vi "TRDU_ADRESSAGE.vi"(8 "errin":errorcluster, 11 "Go?":bool) -> (0 "errout":errorcluster, 2 "Branche":dbl=1.0, 3 "Addressé?":bool)   [LabVIEW 2020]
uses:
  <userlib>/PCAN Basic/Controls/BaudrateEenum.ctl
  <userlib>/PCAN Basic/Controls/Channel.ctl
  OP500/VG/VG_branche.vi
  <userlib>/PCAN Basic/PCANBasic.lvlib
  <userlib>/Alex_Peak_lib/PEAK_lib_ALEX.lvlib
panel:
  out "OBJ":u8[](array[numeric])
  out "CAN":u8[](array[numeric])
  # "READ FROM CAN"
  # "OBJECTIVE TO PASS"
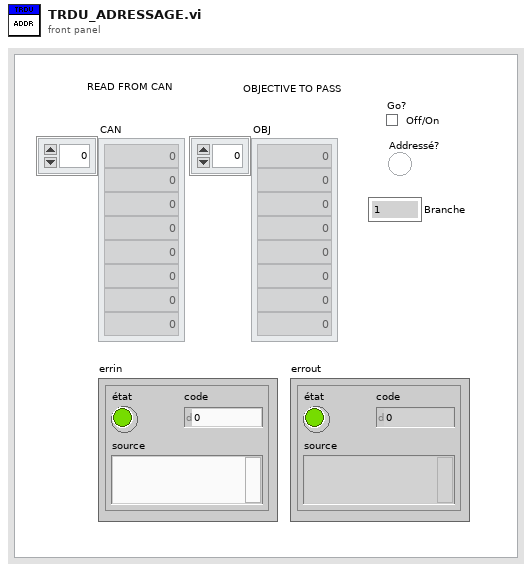
[diagram p1: front panel]
types:
  T1 = typedef "PCANBasic.lvlib/Channel.ctl" = enum16{"PCAN_NONEBUS", "not used1", "not used2", "not used3", "not used4", "not used5", "not used6", "not used7", "not used8", "not used9", "not used10", "not used11", "not used12", "not used13", "not used14", "not used15", "not used16", "not used17", "not used18", "not used19", "not used20", "not used21", "not used22", "not used23", "not used24", "not used25", "not used26", "not used27", "not used28", "not used29", "not used30", "not used31", "not used32", "PCAN_ISABUS1", "PCAN_ISABUS2", "PCAN_ISABUS3", "PCAN_ISABUS4", "PCAN_ISABUS5", "PCAN_ISABUS6", "PCAN_ISABUS7", "PCAN_ISABUS8", "not used41", "not used42", "not used43", "not used44", "not used45", "not used46", "not used47", "not used48", "PCAN_DNGBUS1", "not used50", "not used51", "not used52", "not used53", "not used54", "not used55", "not used56", "not used57", "not used58", "not used59", "not used60", "not used61", "not used62", "not used63", "not used64", "PCAN_PCIBUS1", "PCAN_PCIBUS2", "PCAN_PCIBUS3", "PCAN_PCIBUS4", "PCAN_PCIBUS5", "PCAN_PCIBUS6", "PCAN_PCIBUS7", "PCAN_PCIBUS8", "not used73", "not used74", "not used75", "not used76", "not used77", "not used78", "not used79", "not used80", "PCAN_USBBUS1", "PCAN_USBBUS2", "PCAN_USBBUS3", "PCAN_USBBUS4", "PCAN_USBBUS5", "PCAN_USBBUS6", "PCAN_USBBUS7", "PCAN_USBBUS8", "Not used89", "Not used90", "Not used91", "Not used92", "Not used93", "Not used94", "Not used95", "Not used96", "PCAN_PCCBUS1", "PCAN_PCCBUS2"}
  T2 = typedef "PCANBasic.lvlib/BaudrateEenum.ctl" = enum16{"CAN_Baud_1M", "CAN_Baud_800K", "CAN_BAUD_500K", "CAN_BAUD_250K", "CAN_BAUD_125K", "CAN_BAUD_100K", "CAN_BAUD_95K", "CAN_BAUD_83K", "CAN_BAUD_50K", "CAN_BAUD_47K", "CAN_BAUD_33K", "CAN_BAUD_20K", "CAN_BAUD_10K", "CAN_BAUD_5K", "User Baudrate"}
  T3 = cluster{"ID":u32, "MSGTYPE":u8, "LEN":u8, "DATA[0]":u8, "DATA[1]":u8, "DATA[2]":u8, "DATA[3]":u8, "DATA[4]":u8, "DATA[5]":u8, "DATA[6]":u8, "DATA[7]":u8}
  T4 = cluster{"DATA[0]":u8, "DATA[1]":u8, "DATA[2]":u8, "DATA[3]":u8, "DATA[4]":u8, "DATA[5]":u8, "DATA[6]":u8, "DATA[7]":u8}
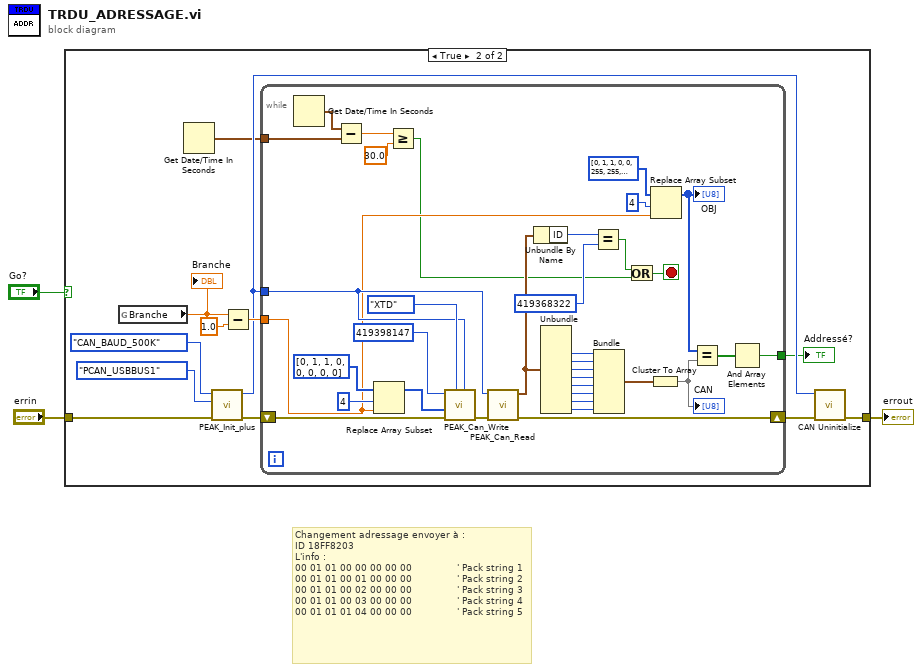
[diagram p0: block diagram]
diagram:
  # "Changement adressage envoyer à :\nID 18FF8203 \nL'info :\n00 01 01 00 00 00 00 00               ' Pack string 1\n00 01 01 00 01 00 00 00               ' Pack string 2\n00 01 01 00 02 00 00 00               ' Pack string 3\n00 01 01 00 03 00 00 00               ' Pack string 4\n00 01 01 01 04 00 00 00               ' Pack string 5"
  n1 = case shown="True" "Go?" {
    tunnel: "errin" -> [w4 w16]
    tunnel: [w4 w8] -> w2
    frame False {
    }
    frame True {
      n2 = global read "VG_branche.vi" "Branche"() -> (w12:dbl)
      "Branche" <- w12
      n3 = Get Date/Time In Seconds() -> (seconds since 1Jan1904=w5:timestamp)
      n4 = call <userlib>:"PEAK_Init_plus.vi"("errin"=w16, "Channel"=Channel."PCAN_USBBUS1", "BTR0BTR1"=BaudrateEenum."CAN_BAUD_500K") -> ("errout"=w13:errorcluster, "Channel out"=w7:T1)  [unwired: 7 in]
      n5 = Subtract(x=w12, y=1.0) -> (x-y=w10:dbl)
      n6 = while {
        tunnel: w10 -> [w38]
        tunnel: w7 -> [w43]
        shift-right: [w44] -> w9
        shift-left: w13 -> [w50]
        tunnel: [w24] -> w6
        tunnel: w5 -> [w20]
        stop <- w22 stop-if-true
        n7 = Get Date/Time In Seconds() -> (seconds since 1Jan1904=w21:timestamp)
        n8 = Subtract(x=w21, y=w20) -> (x-y=w19:dbl)
        n9 = Replace Array Subset(array=u8[] [0, 1, 1, 0, 0, 0, 0, 0] ("CAN Data"), new element=w38, index=4 ("indice")) -> (w45:u8[])
        n10 = Greater Or Equal?(x=w19, y=30.0) -> (x >= y?=w17:bool)
        n11 = call <userlib>:"PEAK_Can_Write.vi"("CAN handle"=w43, "MSG type"=enum8{"STD", "RTR", "XTD", "XTD RTR", "STATUS"}."XTD", "errin"=w50, "CAN Data"=w45, "Identifier"=u32 419398147) -> ("errout"=w49:errorcluster)  [unwired: 6 in]
        n12 = call <userlib>:"PEAK_Can_Read.vi"("errin"=w49, "Channel out"=w43) -> ("errout"=w44:errorcluster, "MessageBuffer out"=w37:T3)  [unwired: 7 in, 1 out]
        n13 = Unbundle By Name(w37) -> ("ID"=w42:u32)
        n14 = Unbundle(w37) -> ("DATA[0]"=w36:u8, "DATA[1]"=w35:u8, "DATA[2]"=w34:u8, "DATA[3]"=w33:u8, "DATA[4]"=w32:u8, "DATA[5]"=w31:u8, "DATA[6]"=w30:u8, "DATA[7]"=w29:u8)  [unwired: 3 out]
        n15 = Equal?(x=w42, y=u32 419368322) -> (x = y?=w23:bool)
        n16 = Bundle("DATA[0]"=w36, "DATA[1]"=w35, "DATA[2]"=w34, "DATA[3]"=w33, "DATA[4]"=w32, "DATA[5]"=w31, "DATA[6]"=w30, "DATA[7]"=w29) -> (w28:T4)  [unwired: 1 in]
        n17 = Or(x=w23, y=w17) -> (x .or. y?=w22:bool)
        n18 = Cluster To Array(cluster=w28) -> (array=w27:u8[])
        "CAN" <- w27
        n19 = Replace Array Subset(array=u8[] [0, 1, 1, 0, 0, 255, 255, 255] ("CAN Data"), new element=w38, index=4 ("indice")) -> (w26:u8[])
        "OBJ" <- w26
        n20 = Equal?(x=w26, y=w27) -> (x = y?=w25:bool[])
        n21 = And Array Elements(Boolean array=w25) -> (logical AND=w24:bool)
      }
      "Addressé?" <- w6
      n22 = call <userlib>:"CAN Uninitialize.vi"("error in (no error)"=w9, "Channel"=w7) -> ("error out"=w8:errorcluster)  [unwired: 7 in, 2 out]
    }
  }
  "errout" <- w2
